vi "Update User.vi"(11 "Username":string) -> ()   [LabVIEW 2020, in "User Lib.lvlib"]
uses:
  User Lib.lvlib
  <vilib>/addons/database/Connection.llb/DB Tools Open Connec (String).vi
  <vilib>/addons/database/NI_Database_API.lvlib
  Database Lib.lvlib
panel:
  out "Error out 3":errorcluster
  out "Error out 2":errorcluster
  in  "Cancel":bool
  in  "OK":bool
  in  "Is Admin?":enum32{"Yes", "No"}(radio)
  in  "Full Name":string
  out "Username 2":string caption="Username"
  # "Update User"
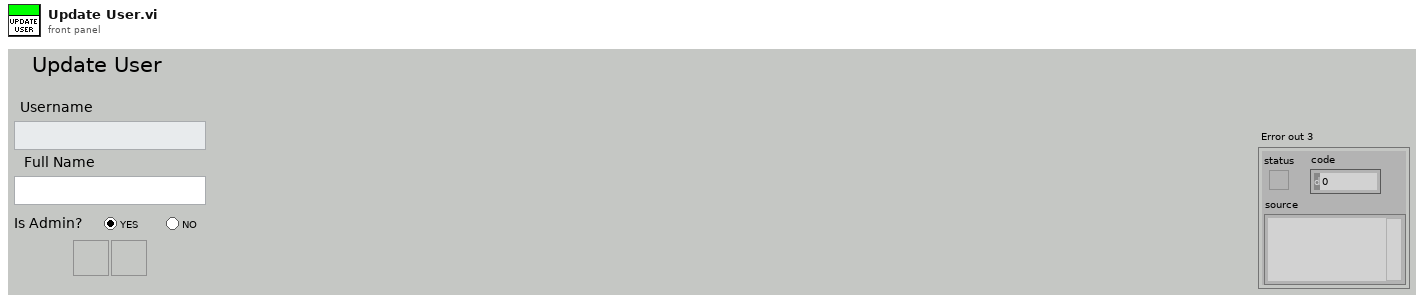
[diagram p1: front panel]
types:
  T1 = cluster{"date/time string":string, "date/time string":string, "code":i32, "date/time string":string, "source":string}
  T2 = typedef "NI_Database_API.lvlib/Conn ObjectReference.ctl" = refnum<k1>
  T3 = cluster{i32, "date/time string":string, "date/time string":string, string}
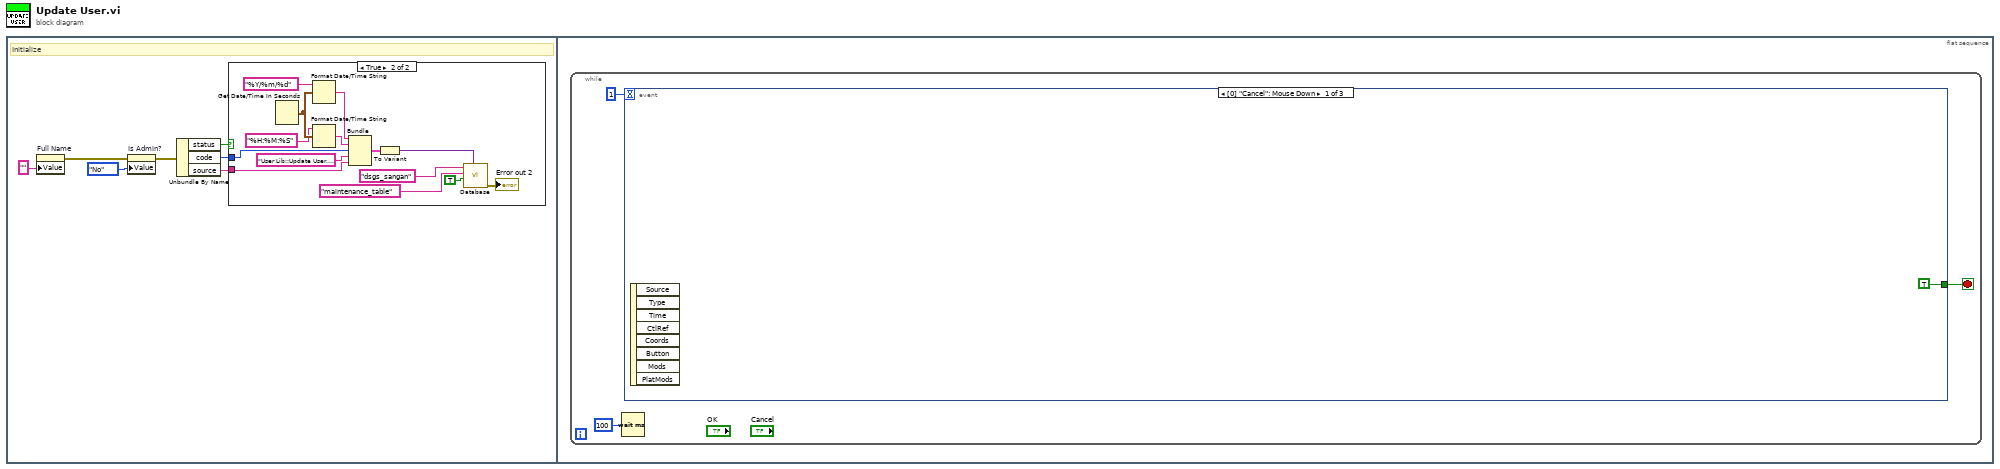
[diagram p0: block diagram]
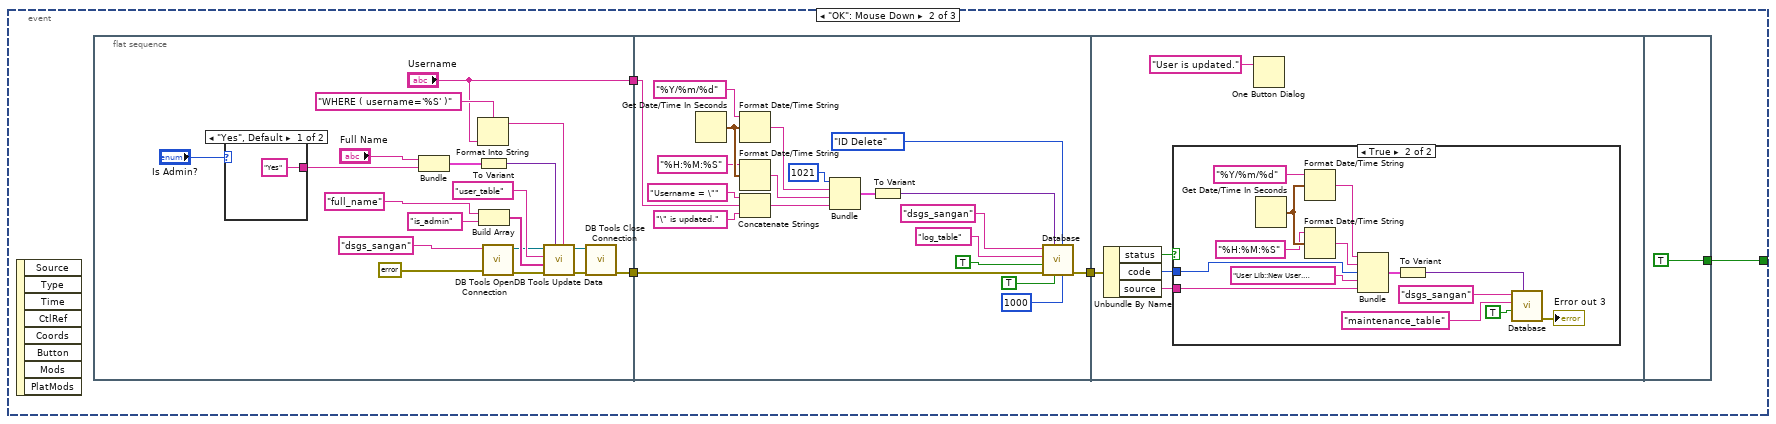
[diagram p3: hidden frame]
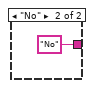
[diagram p4: hidden frame]
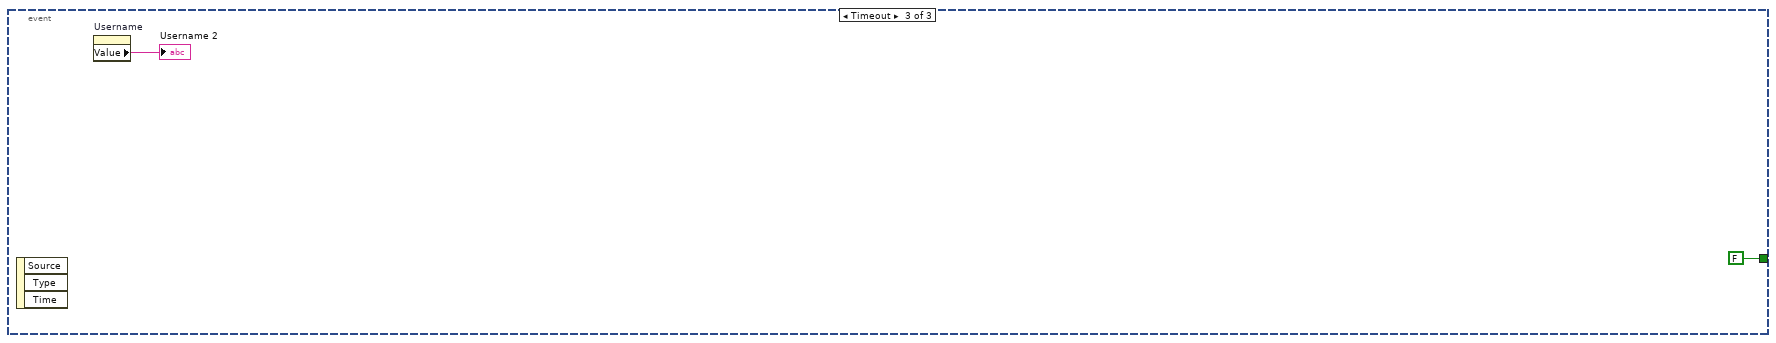
[diagram p6: hidden frame]
diagram:
  n1 = flat-sequence {
    frame #0 {
      # "Initialize"
      n2 = property on="Full Name" class="Str"("Value"="" ("Full Name")) -> (error out=w1:errorcluster)  [unwired: 2 in, 1 out]
      n3 = property on="Is Admin?" class="RadioBtnsControl (strict)"(error in=w1, "Value"=enum32{"Yes", "No"}."No" ("Is Admin?")) -> (error out=w2:errorcluster)  [unwired: 1 in, 1 out]
      n4 = Unbundle By Name(w2) -> ("status"=w4:bool, "code"=w5:i32, "source"=w3:string)
      n5 = case shown="True" w4 {
        tunnel: w5 -> [_ w16]
        tunnel: w3 -> [_ w14]
        frame False {
        }
        frame True {
          n6 = Get Date/Time In Seconds() -> (seconds since 1Jan1904=w21:timestamp)
          n7 = Format Date/Time String(time format string (%c)="%Y/%m/%d", seconds (now)=w21) -> (date/time string=w18:string)  [unwired: 1 in]
          n8 = Format Date/Time String(time format string (%c)="%H:%M:%S", seconds (now)=w21) -> (date/time string=w17:string)  [unwired: 1 in]
          n9 = Bundle("date/time string"=w18, "date/time string"=w17, "code"=w16, "date/time string"="User Lib::Update User.vi::Initialize", "source"=w14) -> (w13:T1)  [unwired: 1 in]
          n10 = To Variant(anything=w13) -> (Variant=w12:variant)
          n11 = call "Database.vi"("Data"=w12, "Auto Increment ID?"=TRUE, "Table"="maintenance_table", "Connection"="dsgs_sangan") -> ("Error out"=→"Error out 2":errorcluster)  [unwired: 7 in]
        }
      }
    }
    frame #1 {
      n12 = while {
        stop <- w24 stop-if-true
        n13 = Wait (ms)(milliseconds to wait=u32 100) -> ()  [unwired: 1 out]
        n14 = event shown="[0] \"Cancel\": Mouse Down" {
          selector: _ -> [_ _ _]
          dyn-events: _ -> [_ _ _]
          timeout: 1 -> [_ _ _]
          tunnel: [TRUE w28 FALSE] -> w24
          event "Cancel": Mouse Down {
            n15 = event-data() -> ()  [unwired: 1 in, 8 out]
          }
          event "OK": Mouse Down {
            n16 = event-data() -> ()  [unwired: 1 in, 8 out]
            n17 = flat-sequence {
              tunnel: [w34] -> w29
              tunnel: ["Username"] -> w27
              tunnel: w29 -> [w56]
              tunnel: w27 -> [w55]
              tunnel: [w52] -> w26
              tunnel: w26 -> [w71]
              tunnel: [TRUE] -> w28
              frame #0 {
                n18 = case shown="\"Yes\", Default" "Is Admin?" {
                  tunnel: ["Yes" ("table") "No" ("table")] -> w45
                  frame "Yes", Default {
                  }
                  frame "No" {
                  }
                }
                n19 = Bundle("Full Name"="Full Name", "table"=w45) -> (w36:cluster{"Full Name":string, "table":string})  [unwired: 1 in]
                n20 = Format Into String(format string="WHERE ( username='%S' )" ("condition"), "Username") -> (resulting string=w41:string)  [unwired: 2 in, 1 out]
                n21 = To Variant(anything=w36) -> (Variant=w35:variant)
                n22 = Build Array("full_name" ("table"), "is_admin" ("table")) -> (w39:string[])
                n23 = call-poly <vilib>:"DB Tools Open Connection.vi"("error in (no error)"=errorcluster {"status"=FALSE, "code"=0, "source"=""}, "connection information"="dsgs_sangan") -> ("error out"=w31:errorcluster, "connection reference"=w32:T2)  [unwired: 6 in]
                n24 = call <vilib>:"DB Tools Update Data.vi"("condition"=w41, "data"=w35, "error in (no error)"=w31, "columns"=w39, "table"="user_table", "connection reference"=w32) -> ("error out"=w43:errorcluster, "connection reference out"=w42:T2)  [unwired: 4 in]
                n25 = call <vilib>:"DB Tools Close Connection.vi"("error in (no error)"=w43, "connection reference"=w42) -> ("error out"=w34:errorcluster)  [unwired: 5 in]
              }
              frame #1 {
                n26 = Get Date/Time In Seconds() -> (seconds since 1Jan1904=w66:timestamp)
                n27 = Format Date/Time String(time format string (%c)="%Y/%m/%d", seconds (now)=w66) -> (date/time string=w67:string)  [unwired: 1 in]
                n28 = Format Date/Time String(time format string (%c)="%H:%M:%S", seconds (now)=w66) -> (date/time string=w68:string)  [unwired: 1 in]
                n29 = Concatenate Strings("Username = \"" ("string"), w55, "\" is updated." ("string")) -> (w65:string)
                n30 = Bundle(1021, "date/time string"=w67, "date/time string"=w68, w65) -> (w69:T3)  [unwired: 1 in]
                n31 = To Variant(anything=w69) -> (Variant=w70:variant)
                n32 = call "Database.vi"("Maximum Row"=1000, "Enum"=enum16{"ID Delete", "Time Delete"}."ID Delete", "Delete row?"=TRUE, "Data"=w70, "Error in"=w56, "Auto Increment ID?"=TRUE, "Table"="log_table" ("table"), "Connection"="dsgs_sangan" ("table")) -> ("Error out"=w52:errorcluster)  [unwired: 3 in]
              }
              frame #2 {
                n33 = Unbundle By Name(w71) -> ("status"=w73:bool, "code"=w74:i32, "source"=w72:string)
                n34 = case shown="True" w73 {
                  tunnel: w74 -> [_ w84]
                  tunnel: w72 -> [_ w82]
                  frame False {
                  }
                  frame True {
                    n35 = Get Date/Time In Seconds() -> (seconds since 1Jan1904=w89:timestamp)
                    n36 = Format Date/Time String(time format string (%c)="%Y/%m/%d", seconds (now)=w89) -> (date/time string=w86:string)  [unwired: 1 in]
                    n37 = Format Date/Time String(time format string (%c)="%H:%M:%S", seconds (now)=w89) -> (date/time string=w85:string)  [unwired: 1 in]
                    n38 = Bundle("date/time string"=w86, "date/time string"=w85, "code"=w84, "date/time string"="User Lib::New User.vi::Initialize", "source"=w82) -> (w81:T1)  [unwired: 1 in]
                    n39 = To Variant(anything=w81) -> (Variant=w80:variant)
                    n40 = call "Database.vi"("Data"=w80, "Auto Increment ID?"=TRUE, "Table"="maintenance_table", "Connection"="dsgs_sangan") -> ("Error out"=→"Error out 3":errorcluster)  [unwired: 7 in]
                  }
                }
                n41 = One Button Dialog(message="User is updated.") -> ()  [unwired: 1 in, 1 out]
              }
              frame #3 {
              }
            }
          }
          event Timeout {
            n42 = event-data() -> ()  [unwired: 1 in, 3 out]
            n43 = property on="Username" class="Str"() -> ("Value"=→"Username 2":string)  [unwired: 2 in, 2 out]
          }
        }
      }
    }
  }
